vi "Convert-U64-Array-to-U32-Array.vi"(11 "2 x U64":u64[](array[numeric])) -> (3 "4 x U32":u32[](array[numeric]))   [LabVIEW 2017]
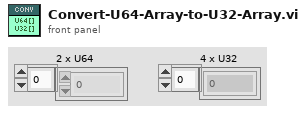
[diagram p1: front panel]
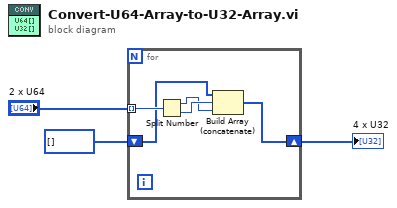
[diagram p0: block diagram]
diagram:
  n1 = for {
    tunnel: "2 x U64" -> [w8] mode=indexing
    shift-right: [w7] -> w2
    shift-left: u32[] [] -> [w6]
    n2 = Split Number(x=w8) -> (hi(x)=w4:u32, lo(x)=w5:u32)
    n3 = Build Array (concatenate)(w6, w5, w4) -> (w7:u32[])
  }
  "4 x U32" <- w2
